vi "ColorText Facade.vi"(0 "Data In":T4, 2 "Display State In":T2, 3 "Container State":T3) -> (6 "Data Out":T4, 7 "Display State Out":T2, 8 "Action":T1)   [LabVIEW 2016, in "Code.xctl"]
uses:
  Code.xctl
  <vilib>/_xctls/Action.ctl
  <vilib>/_xctls/XControlSupport.lvlib
  <vilib>/_xctls/Container State.ctl
  ColorText Data.ctl
  ColorText State.ctl
panel:
  in  "Code":string
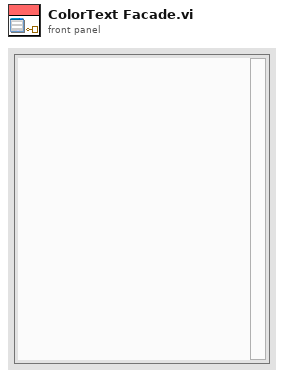
[diagram p1: front panel]
types:
  T1 = typedef "XControlSupport.lvlib/Action.ctl" = cluster{"Data Changed?":bool, "State Changed?":bool, "Action Name":string}
  T2 = typedef "Code.xctl/ColorText State.ctl" = cluster{"Numeric":dbl}
  T3 = typedef "XControlSupport.lvlib/Container State.ctl" = cluster{"Indicator?":bool, "Run Mode?":bool, " Refnum":refnum<vi>}
  T4 = typedef "Code.xctl/ColorText Data.ctl" = string
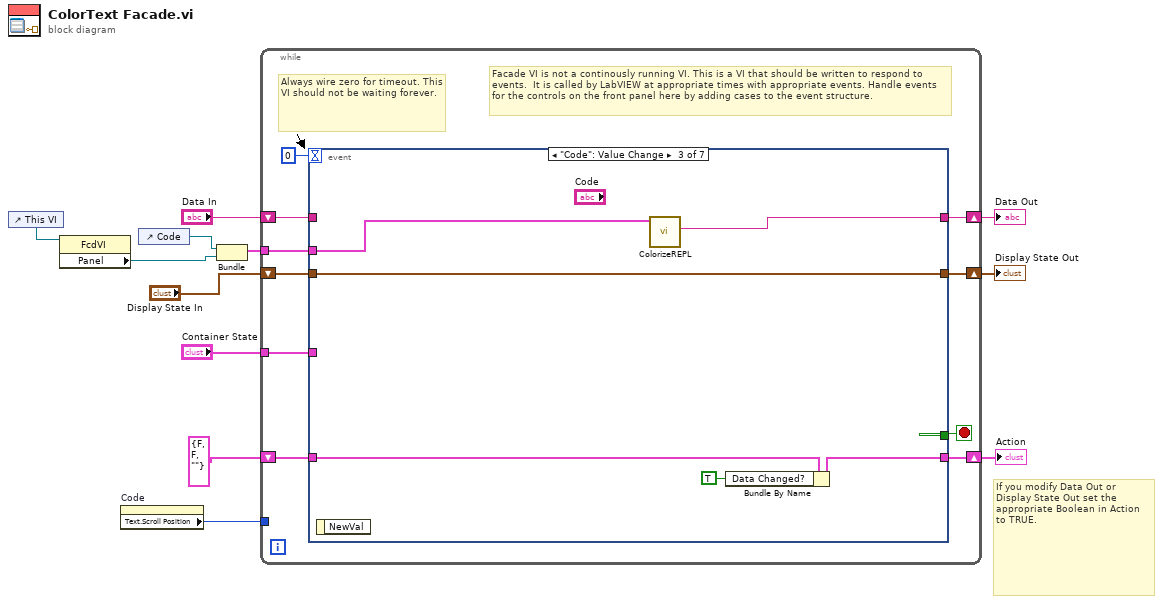
[diagram p0: block diagram]
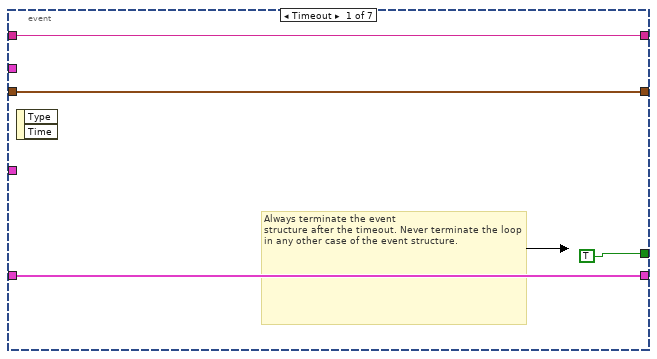
[diagram p2: hidden frame]
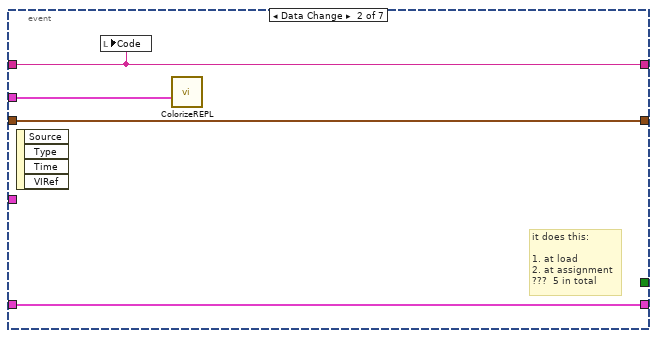
[diagram p3: hidden frame]
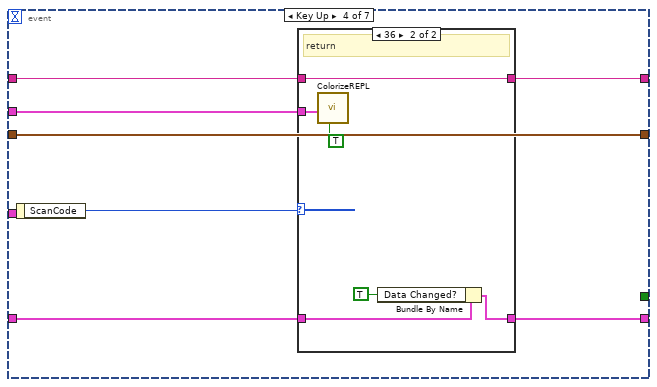
[diagram p4: hidden frame]
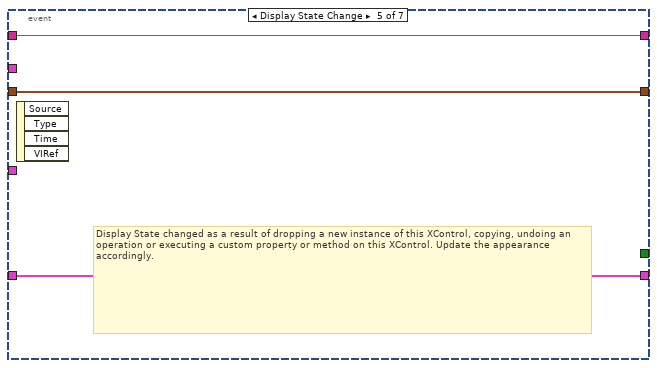
[diagram p6: hidden frame]
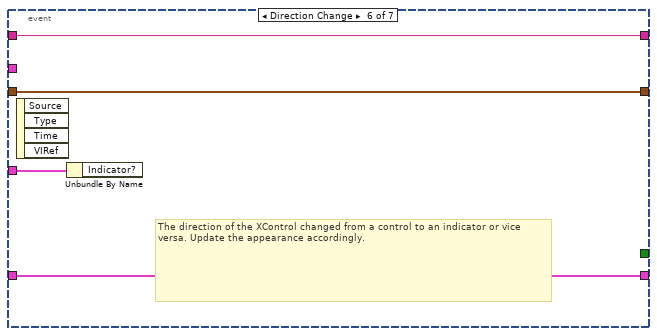
[diagram p7: hidden frame]
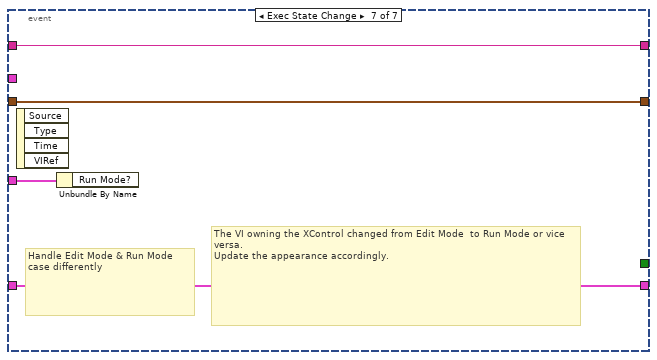
[diagram p8: hidden frame]
diagram:
  # "If you modify Data Out or\nDisplay State Out set the\nappropriate Boolean in Action\nto TRUE."
  n1 = control-ref of="This VI"() -> (w5:refnum<vi>)
  n2 = property class="FcdVI"(reference=w5) -> ("Panel"=w3:refnum<vi>)  [unwired: 1 in, 2 out]
  n3 = property on="Code" class="Str"() -> ("Text.Scroll Position"=w1:u32)  [unwired: 2 in, 2 out]
  n4 = control-ref of="Code"() -> (w2:refnum<vi>)
  n5 = Bundle("Code"=w2, "Panel"=w3) -> (w4:cluster{"Code":refnum<vi>, "Panel":refnum<vi>})  [unwired: 1 in]
  n6 = while {
    shift-right: [w21] -> w9
    shift-left: "Display State In" -> [w22]
    tunnel: "Container State" -> [w19]
    shift-right: [w13] -> w12
    shift-left: "Data In" -> [w18]
    shift-right: [w16] -> w7
    shift-left: T1 {"Data Changed?"=FALSE, "State Changed?"=FALSE, "Action Name"=""} ("Action") -> [w17]
    tunnel: w4 -> [w14]
    tunnel: w1 -> [_]
    stop <- w20 stop-if-true
    # "Facade VI is not a continously running VI. This is a VI that should be written to respond to events.  It is called by LabVIEW at appropriate times with appropriate events. Handle events for the controls on the front panel here by adding cases to the event structure."
    # "Always wire zero for timeout. This\nVI should not be waiting forever."
    n7 = event shown="[2] \"Code\": Value Change" {
      selector: _ -> [_ _ _ _ _ _ _]
      dyn-events: _ -> [_ _ _ _ _ _ _]
      timeout: 0 -> [_ _ _ _ _ _ _]
      tunnel: w22 -> [w24 w30 w36 w43 w54 w57 w61]
      tunnel: [w24 w30 w36 w43 w54 w57 w61] -> w21
      tunnel: [TRUE _ _ _ _ _ _] -> w20
      tunnel: w19 -> [_ _ _ _ _ w58 w62]
      tunnel: w18 -> [w23 w28 _ w39 w52 w55 w59]
      tunnel: [w25 w29 w34 w40 w53 w56 w60] -> w16
      tunnel: w17 -> [w25 w29 w35 w41 w53 w56 w60]
      tunnel: w14 -> [_ w27 w32 w38 _ _ _]
      tunnel: [w23 w28 w31 w37 w52 w55 w59] -> w13
      event Timeout {
        # "Always terminate the event\nstructure after the timeout. Never terminate the loop in any other case of the event structure."
        n8 = event-data() -> ()  [unwired: 1 in, 2 out]
      }
      event Data Change {
        # "it does this:\n\n1. at load\n2. at assignment\n???  5 in total"
        n9 = event-data() -> ()  [unwired: 1 in, 4 out]
        n10 = local write "Code"(w28) -> ()
        n11 = call "ColorizeREPL.vi"("refs"=w27) -> ()  [unwired: 9 in, 1 out]
      }
      event "Code": Value Change {
        n12 = event-data() -> ()  [unwired: 1 in, 1 out]
        n13 = call "ColorizeREPL.vi"("refs"=w32) -> ("Value"=w31:string)  [unwired: 9 in]
        n14 = Bundle By Name(cluster=w35, "Data Changed?"=TRUE) -> (w34:T1)
      }
      event Key Up {
        n15 = event-data() -> ("ScanCode"=w42:i16)  [unwired: 1 in]
        n16 = case shown="36" w42 {
          tunnel: w41 -> [w45 w50]
          tunnel: [w45 w49] -> w40
          tunnel: w39 -> [w44 w46]
          tunnel: [w44 w46] -> w37
          tunnel: w38 -> [_ w47]
          frame Default {
          }
          frame 36 {
            # "return"
            n17 = call "ColorizeREPL.vi"("refs"=w47, "Add Spaces?"=TRUE) -> ()  [unwired: 8 in, 1 out]
            n18 = Bundle By Name(cluster=w50, "Data Changed?"=TRUE) -> (w49:T1)
          }
        }
      }
      event Display State Change {
        # "Display State changed as a result of dropping a new instance of this XControl, copying, undoing an operation or executing a custom property or method on this XControl. Update the appearance accordingly."
        n19 = event-data() -> ()  [unwired: 1 in, 4 out]
      }
      event Direction Change {
        # "The direction of the XControl changed from a control to an indicator or vice versa. Update the appearance accordingly."
        n20 = event-data() -> ()  [unwired: 1 in, 4 out]
        n21 = Unbundle By Name(w58) -> ()  [unwired: 1 out]
      }
      event Exec State Change {
        # "The VI owning the XControl changed from Edit Mode  to Run Mode or vice versa.\nUpdate the appearance accordingly."
        # "Handle Edit Mode & Run Mode\ncase differently"
        n22 = event-data() -> ()  [unwired: 1 in, 4 out]
        n23 = Unbundle By Name(w62) -> ()  [unwired: 1 out]
      }
    }
  }
  "Display State Out" <- w9
  "Data Out" <- w12
  "Action" <- w7
